vi "Create Polynomial From Roots (CDB).vi"(11 "Roots":cdb[](array[numeric]) format="%#.6g") -> (0 "error":i32, 3 "P(x)":cdb[](array[numeric]) format="%#.6g")   [LabVIEW 2010, in "NI_AALPro.lvlib"]
doc: "Creates polynomial <B>P(x)</B> from its roots. Wire data to the <B>Roots</B> input to determine the polymorphic instance to use or manually select the instance."
uses:
  NI_AALPro.lvlib
  Leja Order Roots (CDB).vi
  Multiply Polynomials (DBL).vi
  Multiply Polynomials (CDB).vi
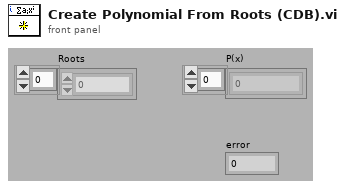
[diagram p1: front panel]
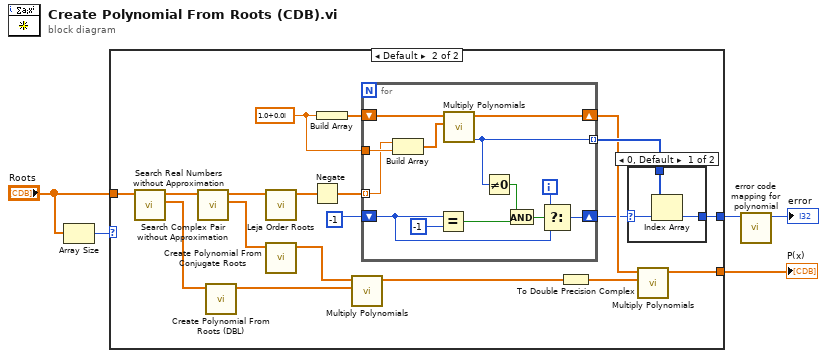
[diagram p0: block diagram]
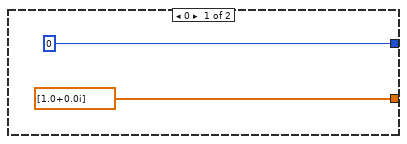
[diagram p2: hidden frame]
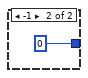
[diagram p3: hidden frame]
diagram:
  n1 = Array Size(array="Roots") -> (size(s)=w4:i32)
  n2 = case shown="Default" w4 {
    tunnel: [cdb[] [1.0+0.0i] ("CDB") w14] -> w5
    tunnel: "Roots" -> [_ w9]
    tunnel: [0 w21] -> w2
    frame 0 {
    }
    frame Default {
      w25 = cdb 1.0+0.0i
      n3 = call "Search Real Numbers without Approximation.vi"("Complex Numbers In"=w9) -> ("Real Numbers"=w19:dbl[], "Complex Numbers Out"=w10:cdb[])  [unwired: 9 in]
      n4 = call "Search Complex Pair without Approximation.vi"("Complex Numbers"=w10) -> ("Complex Pair Numbers"=w20:cdb[], "Pure Complex Numbers"=w12:cdb[])  [unwired: 9 in]
      n5 = call "Create Polynomial From Roots (DBL).vi"("Roots"=w19) -> ("P(x)"=w17:dbl[])  [unwired: 9 in, 1 out]
      n6 = call-poly "Leja Order Roots.vi"("Roots"=w12) -> ("Roots of Leja Order"=w11:cdb[])  [unwired: 10 in]
      n7 = call "Create Polynomial From Conjugate Roots.vi"("Conjugate Complex"=w20) -> ("P(x)"=w18:dbl[])  [unwired: 10 in]
      n8 = Negate(x=w11) -> (-x=w24:cdb[])
      n9 = Build Array(w25) -> (w26:cdb[])
      n10 = call-poly "Multiply Polynomials.vi"("Q(x)"=w17, "P(x)"=w18) -> ("P(x)*Q(x)"=w16:dbl[])  [unwired: 8 in, 1 out]
      n11 = for {
        shift-right: [w32] -> w15
        shift-left: w26 -> [w34]
        tunnel: w25 -> [w43]
        tunnel: w24 -> [w42] mode=indexing
        shift-right: [w35] -> w8
        shift-left: -1 -> [w36]
        tunnel: [w31] -> w22 mode=indexing
        i -> [w38]
        n12 = Build Array(w42, w43) -> (w33:cdb[])
        n13 = Equal?(x=w36, y=-1) -> (x = y?=w39:bool)
        n14 = call-poly "Multiply Polynomials.vi"("Q(x)"=w33, "P(x)"=w34) -> ("error"=w31:i32, "P(x)*Q(x)"=w32:cdb[])  [unwired: 8 in]
        n15 = Not Equal To 0?(x=w31) -> (x != 0?=w40:bool)
        n16 = And(x=w40, y=w39) -> (x .and. y?=w37:bool)
        n17 = Select(t=w38, s=w37, f=w36) -> (s? t:f=w35:i32)
      }
      n18 = To Double Precision Complex(1:w16) -> (0:w13:cdb[])
      n19 = case shown="0, Default" w8 {
        selector: w8 -> [w27 _]
        tunnel: w22 -> [w29 _]
        tunnel: [w28 0 ("error")] -> w21
        frame 0, Default {
          n20 = Index Array(array=w29, index=w27) -> (element=w28:i32)
        }
        frame -1 {
        }
      }
      n21 = call-poly "Multiply Polynomials.vi"("Q(x)"=w13, "P(x)"=w15) -> ("P(x)*Q(x)"=w14:cdb[])  [unwired: 8 in, 1 out]
    }
  }
  "P(x)" <- w5
  n22 = call "error code mapping for polynomial.vi"("error in"=w2) -> ("error out"=→"error":i32)  [unwired: 10 in]
